vi "tpg361_get_p.vi"(8 "err_in":errorcluster, 11 "visa_in":refnum<visa-resource-name>) -> (0 "err_out":errorcluster, 1 "pressure":dbl, 2 "status":i8, 3 "visa_out":refnum<visa-resource-name>, 4 "status_all":bool)   [LabVIEW 2019]
panel:
  out "string":string
  out "status_ack":bool
  out "pressure_str":string
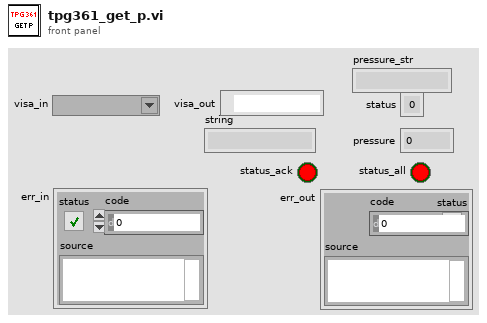
[diagram p1: front panel]
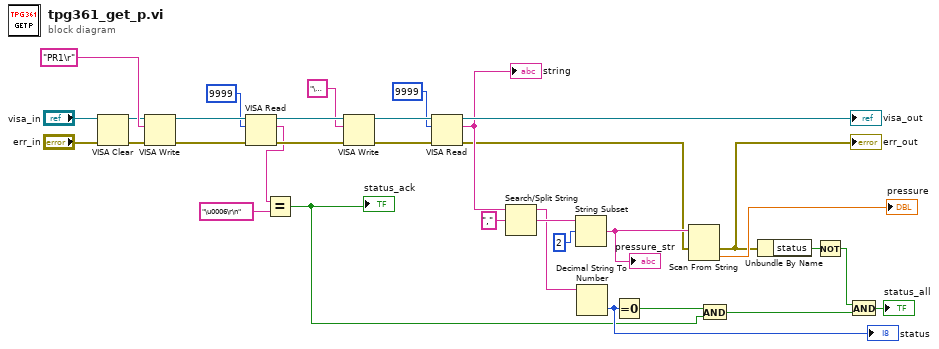
[diagram p0: block diagram]
diagram:
  n1 = VISA Clear(VISA resource name="visa_in", error in (no error)="err_in") -> (VISA resource name out=w14:refnum<visa-resource-name>, error out=w13:errorcluster)
  n2 = VISA Write(VISA resource name=w14, write buffer="PR1\r" ("string"), error in (no error)=w13) -> (VISA resource name out=w33:refnum<visa-resource-name>, error out=w32:errorcluster)  [unwired: 1 out]
  n3 = VISA Read(VISA resource name=w33, byte count=u32 9999, error in (no error)=w32) -> (VISA resource name out=w30:refnum<visa-resource-name>, read buffer=w18:string, error out=w31:errorcluster)  [unwired: 1 out]
  n4 = Equal?(x=w18, y="\u0006\r\n") -> (x = y?=w15:bool)
  "status_ack" <- w15
  n5 = VISA Write(VISA resource name=w30, write buffer="\u0005", error in (no error)=w31) -> (VISA resource name out=w29:refnum<visa-resource-name>, error out=w28:errorcluster)  [unwired: 1 out]
  n6 = VISA Read(VISA resource name=w29, byte count=u32 9999, error in (no error)=w28) -> (VISA resource name out=→"visa_out":refnum<visa-resource-name>, read buffer=w25:string, error out=w4:errorcluster)  [unwired: 1 out]
  "string" <- w25
  n7 = Search/Split String(string=w25, search string/char (-)=",") -> (substring before match=w21:string, match + rest of string=w23:string)  [unwired: 1 in, 1 out]
  n8 = String Subset(string=w23, offset (0)=2) -> (substring=w10:string)  [unwired: 1 in]
  "pressure_str" <- w10
  n9 = Decimal String To Number(string=w21) -> (number=w20:i32)  [unwired: 2 in, 1 out]
  "status" <- w20
  n10 = Equal To 0?(x=w20) -> (x = 0?=w16:bool)
  n11 = Scan From String(input string=w10, error in=w4) -> (error out=w3:errorcluster, output 1=→"pressure":dbl)  [unwired: 3 in, 2 out]
  "err_out" <- w3
  n12 = And(x=w16, y=w15) -> (x .and. y?=w8:bool)
  n13 = Unbundle By Name(w3) -> ("status"=w2:bool)
  n14 = Not(x=w2) -> (.not. x?=w1:bool)
  n15 = And(x=w1, y=w8) -> (x .and. y?=→"status_all":bool)
